vi "Write Header String.vi"(8 "error in (no error)":errorcluster, 10 "Header Contents":T1={"FILENAME"=["FILENAME", "example.fits", "File name at acquisition"], "OBSERVER"=["OBSERVER", "Denis", "Observer’s (PI) name"], "PROGRID"=["PROGRID", "2018A-001", "Program ID"], "OBJECT"=["OBJECT", "UNDEFINED", "Object name"], "NIGHTDIR"=["NIGHTDIR", "DIR", "Night directory name "], "CHANNEL"=["CHANNEL", "RED", "Instrument channel"], "INSTRUME"=["INSTRUME", "ECHARPE", "Instrument"], "NEXPSEQ"=["NEXPSEQ", "1", "Total number of exposures in sequence"], "SEQINDEX"=["SEQINDEX", "1", "Exposure index in the sequence"], "OBSTYPE"=["OBSTYPE", "BIAS", "Image type: OBJECT, BIAS, FLAT, ARC, DARK"], "READMOD"=["READMOD", "Normal", "Read out mode: fast, normal, slow"], "SHUTTER"=["SHUTTER", "CLOSED", "Shutter Mode (OPEN, CLOSED, or AUTO) "], "OPENSHT"=["OPENSHT", "50", "Time to open the shutter (ms) "], "CLOSESHT"=["CLOSESHT", "50", "Time to close the shutter (ms)"], "GAIN"=["GAIN", "3.38", "Gain (e-/ADU)"], "GAINERR "=["GAINERR", "0.05", " Gain error (e-/ADU)"], "RDNOISE"=["RDNOISE", "6.55", "Read noise (e-)"], "RNOISERR"=["RNOISERR", "0.02", "Read noise error (e-)"], "SKYFIBER"=["SKYFIBER", "\"OFF\"", "Sky fiber: ON or OFF"], "CALFIBER"=["CALFIBER", "\"OFF\"", "Calibration Fiber: ON or OFF"], "UTDATE"=["UTDATE", "'2017-10-01T20", "UT date at start of exposure"], "LOCTIME"=["LOCTIME", "'2017-10-01T17", "LT date at start of exposure"], "MJD"=["MJD", "58027.500000", "Modified Julian Date at start of exposure"], "OBSLON"=["OBSLON", "-45.57972", "Observatory East Longitude"], "OBSLAT"=["OBSLAT", "-22.53444", "Observatory Latitude"], "OBSALT"=["OBSALT", "1864.0", "Observatory elevation above sea level (m)"], "EXPTIME"=["EXPTIME", "1", "Exposure time (s)"], "TELRA"=["TELRA", "“00:00:00.000”", "TCS right ascension: “HH:MM:SS.SSS”"], "TELDEC"=["TELDEC", "“+00:00:00.000”", "TCS declination: “+-DD:MM:SS.SSS”"], "RA"=["RA", "“00:00:00.000”", "Requested right Ascension: “HH:MM:SS.SSS”"], "DEC"=["DEC", "“+00:00:00.000”", "Requested Declination: “+- DD:MM:SS.SSS”"], "RA_DEG"=["RA_DEG", "128.84946", "Requested Right Ascension (deg)"], "DEC_DEG"=["DEC_DEG", "+19.648717", "Requested Declination (deg)"], "EPOCH"=["EPOCH", "2000.00", "Epoch for Target coordinates"], "HA"=["HA", "“+01:13:05.98”", "Hour Angle (Sexagesimal)"], "HAD"=["HAD", "1.2183292", "Hour Angle (deg)"], "AIRMASS"=["AIRMASS", "1.085", "Mean airmass for the observation"], "AMSTART"=["AMSTART", "1.060", "Airmass at start of exposure"], "AMEND"=["AMEND", "1.114", "Airmass at end of exposure"], "XOFFSET"=["XOFFSET", "0.000000", "Telescope RA offset in arcsec"], "YOFFSET"=["YOFFSET", "0.000000", "Telescope DEC offset in arcsec"], "PA"=["PA", "14.6415392418", "Current Rotator Position Angle (degree)"], "CAMFOC"=["CAMFOC", "-3.53", "Camera focus position (mm)"], "TELFOC"=["TELFOC", "-3.53", "Telescope focus position (mm)"], "TCSUT"=["TCSUT", "‘23:17:24.8’", "TCS Universal Time"], "MOONDIST"=["MOONDIST", "60.0", "Moon angular distance to object (deg)"], "MOONALT"=["MOONALT", "15.0", "Moon elevation above horizon (deg)"], "MONNPHAS"=["MOONPHAS", "30.0", "Moon phase (deg)"], "ADC"=["ADC", "\"ON\"", "Atmospheric Dispersion Corrector: ON or OFF"], "ADCSPPED"=["ADCSPPED", "5.0", "ADC motor speed (rpm)"], "CALMIRR"=["CALMIRR", "\"OUT\"", "Calibration mirror position: IN or OUT"], "GUIDING"=["GUIDING", "“ON”", "Guider status: ON or OFF"], "GUIDTEXP"=["GUIDTEXP", "1.0", "Guider exposure time (s)"], "GUIDFREQ"=["GUIDFREQ", "1.0", "Guiding frequency (Hz)"], "GUIDOBJX"=["GUIDOBJX", "102.5", "Guiding object x position (pixel)"], "GUIDOBJY"=["GUIDOBJY", "300.3", "Guiding object y position (pixel)"], "AVGYCORR"=["AVGYCORR", "2.3", "Average correction in RA (arcsec)"], "AVGXCORR"=["AVGXCORR", "1.3", "Average correction in DEC (arcsec)"], "GFOCUS"=["GFOCUS", "3.0", "Guider focus position (mm)"], "THARLAMP"=["THARLAMP", "“OFF”", "Thorium-Argon lamp state: ON or OFF"], "HALLAMP"=["HALLAMP", "“OFF”", "Halogen lamp state: ON or OFF"], "AGITATOR"=["AGITATOR", "“ON”", "Fiber agitator: ON or OFF"], "THARMIRR"=["THARMIRR", "“SPECTROGRAPH”", "Th-Ar mirror position: SPECTROGRAPH or TELESCOPE"], "DSTATUS"=["DSTATUS", "‘OPEN’", "Dome Status: OPEN or CLOSED"], "DTEMP"=["DTEMP", "10.0", "Dome temperature (deg C)"], "DHUM"=["DHUM", "82.0", "Dome humidity (per cent)"], "DLAMP"=["DLAMP", "“OFF”", "Dome lamp: ON or OFF"], "DFLAT"=["DFLAT", "“OFF”", "Dome flat lamp: ON or OFF"], "TEMPEXT"=["TEMPEXT", "10.0", "External temperature (deg C)"], "PRESSURE"=["PRESSURE", "742.00", "Pressure (mbar)"], "HUMIDITY"=["HUMIDITY", "92.00", "Humidity (per cent)"], "WINDDIR"=["WINDDIR", "15.0", "Wind direction: North-eastward (deg)"], "WSPEED"=["WSPEED", "30.2", "Wind Speed (km/h)"], "TCSST"=["TCSST", "‘23:12:32.5’", "TCS Sideral Time"], "DPOS"=["DPOS", "0.00000", "Dome position (deg)"]}, 11 "RxTxCamera in":refnum<class "RxTxCamera.lvclass">) -> (0 "error out":errorcluster, 3 "RxTxCamera out":refnum<class "RxTxCamera.lvclass">)   [LabVIEW 2018, in "RxTxCamera.lvclass"]
doc: "Este VI recebe um cluster contendo as informações do header e constrói a string do hedaer com a tag HEADER na primeira linha."
uses:
  RxTxCamera.lvclass
  C:/Users/Cliente/Desktop/Software Echarpe/RxTx/RxTx.lvclass
  RxTxCamera.lvclass/RxTxCamera.ctl
  Construct String Header/Construct String Header.lvclass/Construct String Header.ctl
  RxTx/RxTx.lvclass/RxTx.ctl
  Construct String Header/Construct String Header.lvclass
  RxTx/RxTx.lvclass
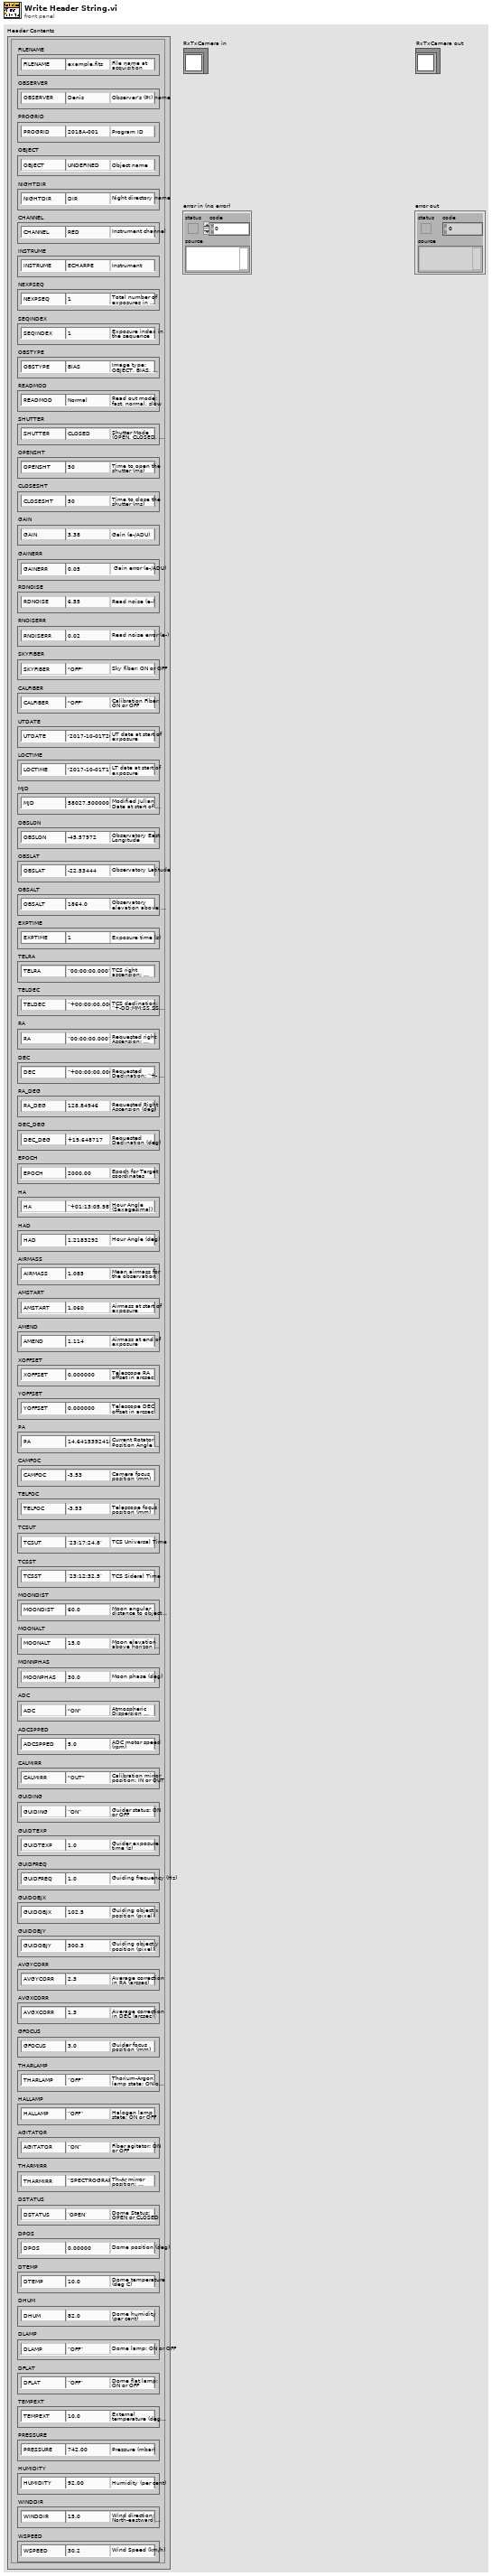
[diagram p1: front panel]
types:
  T1 = cluster{"FILENAME":string[], "OBSERVER":string[], "PROGRID":string[], "OBJECT":string[], "NIGHTDIR":string[], "CHANNEL":string[], "INSTRUME":string[], "NEXPSEQ":string[], "SEQINDEX":string[], "OBSTYPE":string[], "READMOD":string[], "SHUTTER":string[], "OPENSHT":string[], "CLOSESHT":string[], "GAIN":string[], "GAINERR ":string[], "RDNOISE":string[], "RNOISERR":string[], "SKYFIBER":string[], "CALFIBER":string[], "UTDATE":string[], "LOCTIME":string[], "MJD":string[], "OBSLON":string[], "OBSLAT":string[], "OBSALT":string[], "EXPTIME":string[], "TELRA":string[], "TELDEC":string[], "RA":string[], "DEC":string[], "RA_DEG":string[], "DEC_DEG":string[], "EPOCH":string[], "HA":string[], "HAD":string[], "AIRMASS":string[], "AMSTART":string[], "AMEND":string[], "XOFFSET":string[], "YOFFSET":string[], "PA":string[], "CAMFOC":string[], "TELFOC":string[], "TCSUT":string[], "MOONDIST":string[], "MOONALT":string[], "MONNPHAS":string[], "ADC":string[], "ADCSPPED":string[], "CALMIRR":string[], "GUIDING":string[], "GUIDTEXP":string[], "GUIDFREQ":string[], "GUIDOBJX":string[], "GUIDOBJY":string[], "AVGYCORR":string[], "AVGXCORR":string[], "GFOCUS":string[], "THARLAMP":string[], "HALLAMP":string[], "AGITATOR":string[], "THARMIRR":string[], "DSTATUS":string[], "DTEMP":string[], "DHUM":string[], "DLAMP":string[], "DFLAT":string[], "TEMPEXT":string[], "PRESSURE":string[], "HUMIDITY":string[], "WINDDIR":string[], "WSPEED":string[], "TCSST":string[], "DPOS":string[]}
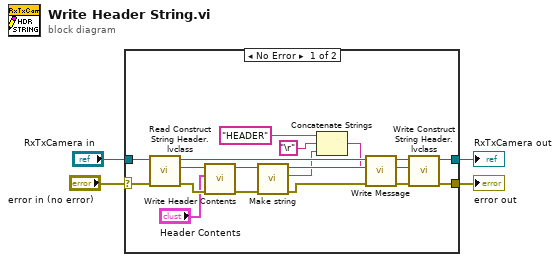
[diagram p0: block diagram]
diagram:
  n1 = case shown="No Error" "error in (no error)" {
    selector: "error in (no error)" -> [w5 w23]
    tunnel: [w21 w23] -> w3
    tunnel: [w22 w24] -> w1
    tunnel: "RxTxCamera in" -> [w6 w24]
    frame No Error {
      n2 = call "Read Construct String Header.lvclass.vi"("error in (no error)"=w5, "RxTxCamera in"=w6) -> ("error out"=w20:errorcluster, "Construct String Header.lvclass"=w19:refnum<class "Construct String Header.lvclass">, "RxTxCamera out"=w12:refnum<class "RxTxCamera.lvclass">)  [unwired: 7 in]
      n3 = call "Write Header Contents.vi"("error in (no error)"=w20, "Header Contents"="Header Contents", "Construct String Header in"=w19) -> ("error out"=w18:errorcluster, "Construct String Header out"=w16:refnum<class "Construct String Header.lvclass">)  [unwired: 7 in]
      n4 = call "Make string.vi"("error in (no error)"=w18, "Construct String Header in"=w16) -> ("error out"=w11:errorcluster, "String Header"=w9:string, "Construct String Header out"=w17:refnum<class "Construct String Header.lvclass">)  [unwired: 7 in]
      n5 = Concatenate Strings("HEADER", "\r", w9) -> (w10:string)
      n6 = call "Write Message.vi"("error in (no error)"=w11, "Message"=w10, "RxTx in"=w12) -> ("error out"=w14:errorcluster, "RxTx out"=w13:refnum<class "RxTxCamera.lvclass">)  [unwired: 7 in]
      n7 = call "Write Construct String Header.lvclass.vi"("error in (no error)"=w14, "Construct String Header.lvclass"=w17, "RxTxCamera in"=w13) -> ("error out"=w21:errorcluster, "RxTxCamera out"=w22:refnum<class "RxTxCamera.lvclass">)  [unwired: 7 in]
    }
    frame Error {
    }
  }
  "error out" <- w3
  "RxTxCamera out" <- w1
